vi "Write to TDMS.vi"() -> ()   [LabVIEW 2014]
uses:
  Formula Hybrid 2012 r1/FPGA Telem for Slow Logging.ctl
  Formula Hybrid 2012 r1/Global Data.vi
panel:
  out "size(s)":i32[](array[numeric])
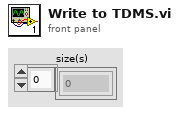
[diagram p1: front panel]
types:
  T1 = enum16{"open", "open or create", "create or replace", "create", "open (read-only)"}
  T2 = cluster{"read mode":enum16{"polling", "blocking"}, "write mode":enum16{"polling", "blocking"}}
  T3 = typedef "FPGA Telem for Slow Logging.ctl" = cluster{"TSBRIO":fxp<+/-,16,9>, "VsbRIOSpply":fxp<+/-,25,6>, "bFPGALED":bool, "CPU Load":cluster{"Total (%)":dbl, "Time Critical (%)":dbl, "Timed Structures (%)":dbl, "High (%)":dbl, "Above Normal (%)":dbl, "Normal (%)":dbl, "Background (%)":dbl, "Idle (%)":dbl, "ISR (%)":dbl}, "Time Stamp":timestamp, "NLatiPhone":dbl, "NLongiPhone":dbl, "nGPSiPhone":dbl, "IHighCurrent":fxp<+/-,24,15>, "ILowCurrent":fxp<+/-,24,15>, "V5VSupply":fxp<+/-,24,5>, "tCurrentLap":u32, "tLastLap":u32, "NLap":u8, "bCoolantPumpEnable":bool, "bRTDSEnable":bool, "bTSMSInStatus":bool, "bPosAIREnable":bool, "bBMSOK":bool, "bIMDOK":bool, "bBSPDOK":bool, "bSBRIOOK2":bool, "bSBRIOOK1":bool, "bTSMSOutStatus":bool, "bMotorControllerEnable":bool, "Tire Diameter(m)":fxp<+,16,1>}
  T4 = cluster{"Total (%)":dbl, "Time Critical (%)":dbl, "Timed Structures (%)":dbl, "High (%)":dbl, "Above Normal (%)":dbl, "Normal (%)":dbl, "Background (%)":dbl, "Idle (%)":dbl, "ISR (%)":dbl}
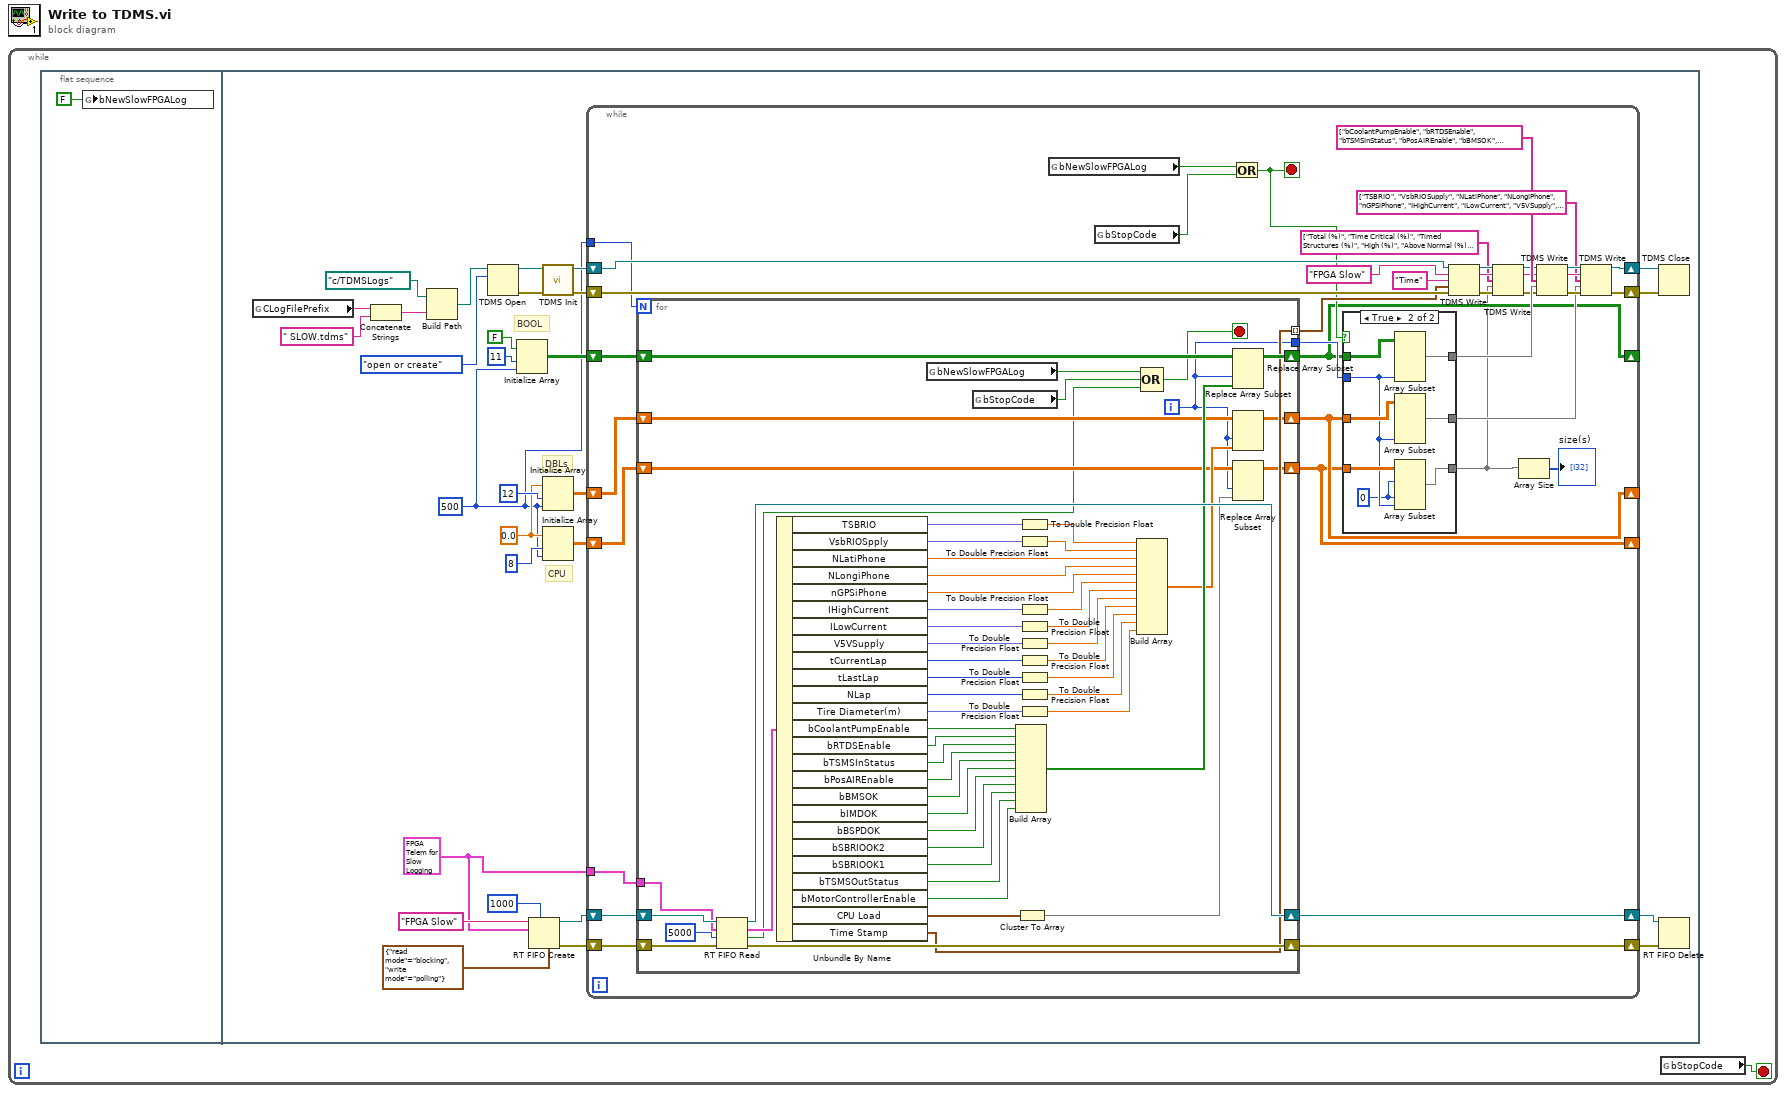
[diagram p0: block diagram]
diagram:
  n1 = while {
    stop <- w1 stop-if-true
    n2 = flat-sequence {
      frame #0 {
        n3 = global write "Global Data.vi" "bNewSlowFPGALog"(FALSE ("New S_FPGA TDMS")) -> ()
      }
      frame #1 {
        w9 = 0.0 ("Total (%)")
        w6 = 500 ("dimension size")
        w26 = T3 {"TSBRIO"=0.0, "VsbRIOSpply"=0.0, "bFPGALED"=FALSE, "CPU Load"={"Total (%)"=0.0, "Time Critical (%)"=0.0, "Timed Structures (%)"=0.0, "High (%)"=0.0, "Above Normal (%)"=0.0, "Normal (%)"=0.0, "Background (%)"=0.0, "Idle (%)"=0.0, "ISR (%)"=0.0}, "Time Stamp"=timestamp(0 s since 1904-01-01), "NLatiPhone"=0.0, "NLongiPhone"=0.0, "nGPSiPhone"=0.0, "IHighCurrent"=0.0, "ILowCurrent"=0.0, "V5VSupply"=-16.0, "tCurrentLap"=4, "tLastLap"=0, "NLap"=0, "bCoolantPumpEnable"=FALSE, "bRTDSEnable"=FALSE, "bTSMSInStatus"=FALSE, "bPosAIREnable"=FALSE, "bBMSOK"=TRUE, "bIMDOK"=TRUE, "bBSPDOK"=FALSE, "bSBRIOOK2"=FALSE, "bSBRIOOK1"=FALSE, "bTSMSOutStatus"=FALSE, "bMotorControllerEnable"=FALSE, "Tire Diameter(m)"=0.0} ("FPGA Logging Telem")
        # "CPU"
        # "BOOL"
        # "DBLs"
        n4 = global read "Global Data.vi" "CLogFilePrefix"() -> (w5:string)
        n5 = Concatenate Strings(w5, " SLOW.tdms" ("string")) -> (w3:string)
        n6 = Build Path(base path=path "c:/TDMSLogs", name or relative path=w3) -> (appended path=w25:path)
        n7 = TDMS Open(10:T1."open or create" ("operation (0:open)"), 11:w25) -> (0:w19:errorcluster, 3:w20:refnum<k34>)  [unwired: 5 in]
        n8 = Initialize Array(FALSE ("Brake Light Out"), 11 ("dimension size"), w6) -> (w11:bool[][])
        n9 = RT FIFO Create(0:"FPGA Slow" ("name (unnamed)"), 1:w26, 4:u32 1000 ("size (10)"), 7:T2 {"read mode"=enum."blocking", "write mode"=enum."polling"} ("r/w modes (polling,polling)")) -> (8:w28:refnum<k33>, 11:w27:errorcluster)  [unwired: 4 in, 1 out]
        n10 = call "TDMS Init.vi"("error in (no error)"=w19, "tdms file"=w20) -> ("error out"=w17:errorcluster, "tdms file out"=w18:refnum<k34>)  [unwired: 8 in]
        n11 = Initialize Array(w9, 12 ("dimension size"), w6) -> (w10:dbl[][])
        n12 = Initialize Array(w9, 8 ("dimension size"), w6) -> (w7:dbl[][])
        n13 = while {
          tunnel: w26 -> [w68]
          shift-right: [w67] -> w15
          shift-left: w28 -> [w70]
          shift-right: [w66] -> w16
          shift-left: w27 -> [w69]
          shift-right: [w53] -> w22
          shift-left: w18 -> [w65]
          shift-right: [w52] -> w21
          shift-left: w17 -> [w64]
          shift-right: [w40] -> _
          shift-left: w11 -> [w51]
          shift-right: [w39] -> _
          shift-left: w10 -> [w48]
          shift-right: [w38] -> _
          shift-left: w7 -> [w47]
          tunnel: w6 -> [w37]
          stop <- w44 stop-if-true
          n14 = for {
            N: w37 -> [_]
            tunnel: w68 -> [w134]
            shift-right: [w132] -> w67
            shift-left: w70 -> [w136]
            shift-right: [w131] -> w66
            shift-left: w69 -> [w135]
            shift-right: [w112] -> w40
            shift-left: w51 -> [w114]
            tunnel: [w111] -> w50 mode=indexing
            shift-right: [w108] -> w39
            shift-left: w48 -> [w110]
            shift-right: [w104] -> w38
            shift-left: w47 -> [w105]
            tunnel: [w103] -> w43
            i -> [w103]
            stop <- w99 stop-if-true
            n15 = RT FIFO Read(0:w136, 1:w134, 2:5000 ("timeout in ms (0)"), 3:w135) -> (8:w132:refnum<k33>, 9:w130:T3, 10:w100:bool, 11:w131:errorcluster)  [unwired: 1 out]
            n16 = Unbundle By Name(w130) -> ("TSBRIO"=w129:fxp<+/-,16,9>, "VsbRIOSpply"=w128:fxp<+/-,25,6>, "NLatiPhone"=w98:dbl, "NLongiPhone"=w97:dbl, "nGPSiPhone"=w96:dbl, "IHighCurrent"=w95:fxp<+/-,24,15>, "ILowCurrent"=w94:fxp<+/-,24,15>, "V5VSupply"=w91:fxp<+/-,24,5>, "tCurrentLap"=w89:u32, "tLastLap"=w88:u32, "NLap"=w87:u8, "Tire Diameter(m)"=w83:fxp<+,16,1>, "bCoolantPumpEnable"=w125:bool, "bRTDSEnable"=w124:bool, "bTSMSInStatus"=w123:bool, "bPosAIREnable"=w122:bool, "bBMSOK"=w121:bool, "bIMDOK"=w120:bool, "bBSPDOK"=w119:bool, "bSBRIOOK2"=w118:bool, "bSBRIOOK1"=w117:bool, "bTSMSOutStatus"=w116:bool, "bMotorControllerEnable"=w115:bool, "CPU Load"=w107:T4, "Time Stamp"=w111:timestamp)
            n17 = global read "Global Data.vi" "bNewSlowFPGALog"() -> (w102:bool)
            n18 = global read "Global Data.vi" "bStopCode"() -> (w101:bool)
            n19 = Build Array(w125, w124, w123, w122, w121, w120, w119, w118, w117, w116, w115) -> (w113:bool[])
            n20 = Cluster To Array(cluster=w107) -> (array=w106:dbl[])
            n21 = To Double Precision Float(number=w129) -> (double precision float=w127:dbl)
            n22 = To Double Precision Float(number=w128) -> (double precision float=w126:dbl)
            n23 = To Double Precision Float(number=w95) -> (double precision float=w93:dbl)
            n24 = To Double Precision Float(number=w94) -> (double precision float=w92:dbl)
            n25 = To Double Precision Float(number=w91) -> (double precision float=w90:dbl)
            n26 = To Double Precision Float(number=w89) -> (double precision float=w86:dbl)
            n27 = To Double Precision Float(number=w88) -> (double precision float=w85:dbl)
            n28 = To Double Precision Float(number=w87) -> (double precision float=w84:dbl)
            n29 = To Double Precision Float(number=w83) -> (double precision float=w82:dbl)
            n30 = Build Array(w127, w126, w98, w97, w96, w93, w92, w90, w86, w85, w84, w82) -> (w109:dbl[])
            n31 = Compound Arithmetic op=OR(w102, w101, w100) -> (w99:bool)
            n32 = Replace Array Subset(array=w114, new element=w113, index (col)=w103) -> (w112:bool[][])  [unwired: 1 in]
            n33 = Replace Array Subset(array=w110, new element=w109, index (col)=w103) -> (w108:dbl[][])  [unwired: 1 in]
            n34 = Replace Array Subset(array=w105, new element=w106, index (col)=w103) -> (w104:dbl[][])  [unwired: 1 in]
          }
          n35 = global read "Global Data.vi" "bNewSlowFPGALog"() -> (w45:bool)
          n36 = global read "Global Data.vi" "bStopCode"() -> (w46:bool)
          n37 = Or(x=w45, y=w46) -> (x .or. y?=w44:bool)
          n38 = case shown="True" w44 {
            tunnel: w38 -> [w73 w81]
            tunnel: w40 -> [w72 w80]
            tunnel: w39 -> [w71 w79]
            tunnel: w43 -> [_ w78]
            tunnel: [w73 w77] -> w33
            tunnel: [w72 w76] -> w42
            tunnel: [w71 w75] -> w41
            frame False {
            }
            frame True {
              w74 = 0 ("index")
              n39 = Array Subset(array=w80, length (col)=w78) -> (w76:bool[][])  [unwired: 3 in]
              n40 = Array Subset(array=w79, length (col)=w78) -> (w75:dbl[][])  [unwired: 3 in]
              n41 = Array Subset(array=w81, index (row)=w74, index (col)=w74, length (col)=w78) -> (w77:dbl[][])  [unwired: 1 in]
            }
          }
          n42 = TDMS Write(0:w65, 5:"FPGA Slow" ("group name in (Untitled)"), 7:"Time", 9:w50, 11:w64) -> (4:w62:refnum<k34>, 6:w60:string, 15:w61:errorcluster)  [unwired: 1 in, 1 out]
          n43 = TDMS Write(0:w62, 5:w60, 7:string[] ["Total (%)", "Time Critical (%)", "Timed Structures (%)", "High (%)", "Above Normal (%)", "Normal (%)", "Background (%)", "Idle (%)", "ISR (%)"] ("channel name(s) in (Untitled)"), 9:w33, 11:w61) -> (4:w36:refnum<k34>, 6:w35:string, 15:w34:errorcluster)  [unwired: 1 in, 1 out]
          n44 = Array Size(array=w33) -> (size(s)=→"size(s)":i32[])
          n45 = TDMS Write(0:w36, 5:w35, 7:string[] ["bCoolantPumpEnable", "bRTDSEnable", "bTSMSInStatus", "bPosAIREnable", "bBMSOK", "bIMDOK", "bBSPDOK", "bSBRIOOK2", "bSBRIOOK1", "bTSMSOutStatus", "bMotorControllerEnable", "BSPD In", "Brake Light Out"] ("channel name(s) in (Untitled)"), 9:w42, 11:w34) -> (4:w57:refnum<k34>, 6:w55:string, 15:w56:errorcluster)  [unwired: 1 in, 1 out]
          n46 = TDMS Write(0:w57, 5:w55, 7:string[] ["TSBRIO", "VsbRIOSupply", "NLatiPhone", "NLongiPhone", "nGPSiPhone", "IHighCurrent", "ILowCurrent", "V5VSupply", "tCurrentLap", "tLastLap", "NLap", "Tire Diameter(m)"] ("channel name(s) in (Untitled)"), 9:w41, 11:w56) -> (4:w53:refnum<k34>, 15:w52:errorcluster)  [unwired: 1 in, 2 out]
        }
        n47 = TDMS Close(8:w21, 11:w22) -> ()  [unwired: 2 out]
        n48 = RT FIFO Delete(0:w15, 3:w16) -> ()  [unwired: 1 in, 1 out]
      }
    }
    n49 = global read "Global Data.vi" "bStopCode"() -> (w1:bool)
  }
